vi "Demo - Transient Capture (Multiple Shots)_for_sub_panel.vi"(6 "Soft Trigger":bool=TRUE, 9 "Post-Trigger Samples":i32=100000, 10 "Pre-Trigger Samples":i32, 11 "configuration file path":path) -> ()   [LabVIEW 2017]
doc: "Demonstration of transient capture mode, in a continuos loop"
uses:
  Communications/Communications Library.lvlib
panel:
  in  "stop":bool
  in  "ARM":bool
  out "Waveform Graph":i16[][](graph)
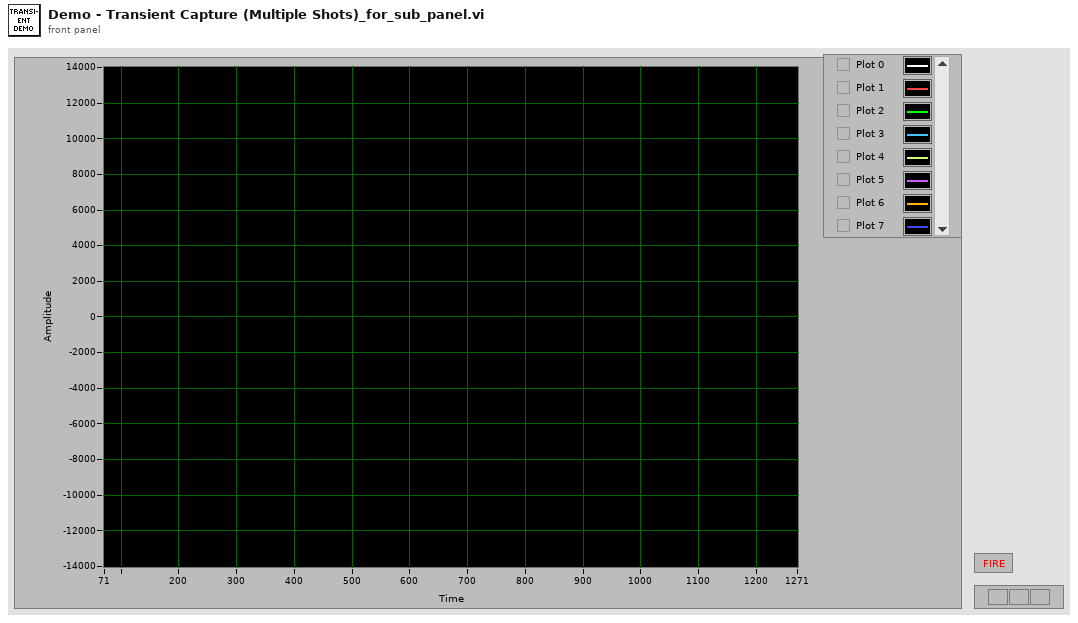
[diagram p1: front panel]
types:
  T1 = typedef "Communications Library.lvlib/DTACQ Module Carrier Configuration--Cluster.ctl" = cluster{"Name":string, "IP":string, "Control Port":i32, "Timeout (ms)":i32, "Continuous Capture Port (Multiplexed)":i32, "Start HIL Shot Port":i32, "AWG Upload Port (Multiplexed)":i32, "Download Captured Data Port (Multiplexed)":i32, "Module Slots":i32, "Module Configurations":T2[]}
  T2 = typedef "Communications Library.lvlib/DTACQ Module Configuration--Cluster.ctl" = cluster{"Name":string, "Position":string, "Module Type":T3, "Control Port":i32, "Timeout (ms)":i32, "Channels":i32}
  T3 = typedef "Communications Library.lvlib/DTACQ Device Type--Enum.ctl" = enum16{"Carrier", "Analog In Module", "Analog Out Module", "Generic Module"}
  T4 = typedef "Communications Library.lvlib/DTACQ Connection Data--Cluster.ctl" = cluster{"Description":string, "Address":string, "Port":u16, "timeout (ms)":i32, "Termination Character":string, "TCP Connection Reference":refnum<k5>, "Open Connection":bool}
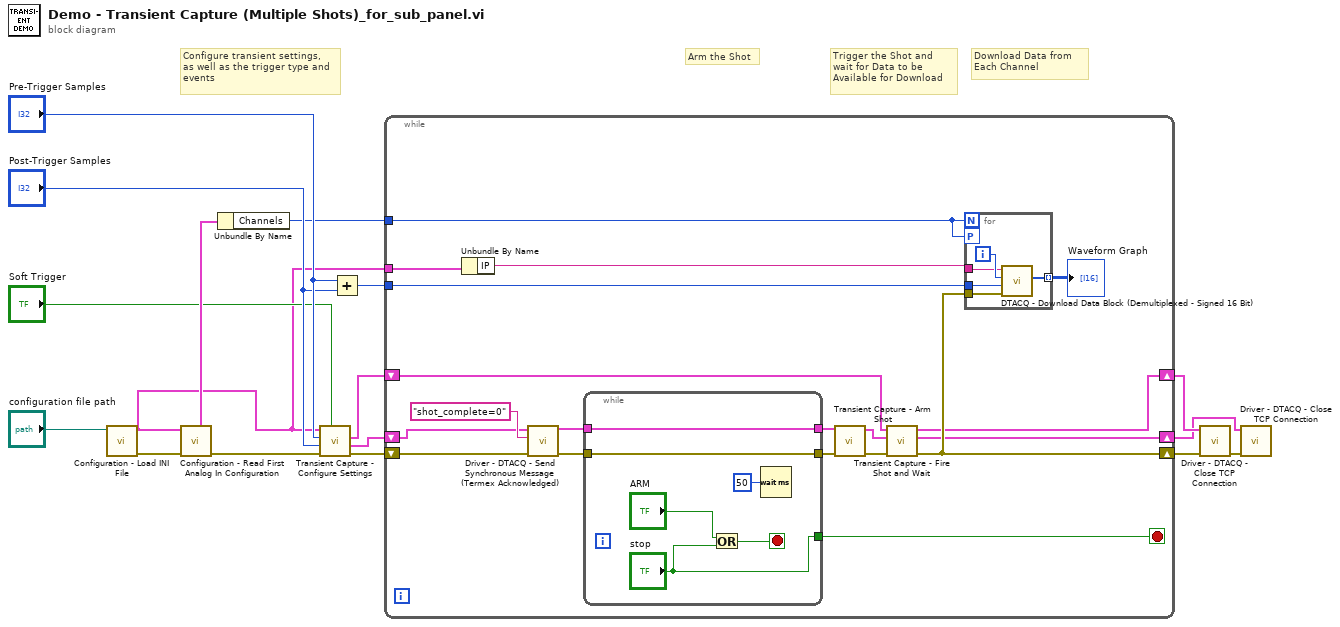
[diagram p0: block diagram]
diagram:
  # "Configure transient settings,\nas well as the trigger type and\nevents"
  # "Trigger the Shot and\nwait for Data to be\nAvailable for Download"
  # "Download Data from \nEach Channel"
  # "Arm the Shot"
  n1 = call "Configuration - Load INI File.vi"("configuration file path"="configuration file path") -> ("error out"=w13:errorcluster, "Carrier Configuration Out"=w1:T1)  [unwired: 9 in]
  n2 = call "Configuration - Read First Analog In Configuration.vi"("error in"=w13, "Carrier Configuration"=w1) -> ("error out"=w12:errorcluster, "AI - Module Configuration"=w14:T2)  [unwired: 5 in, 3 out]
  n3 = Unbundle By Name(w14) -> ("Channels"=w4:i32)
  n4 = call "Transient Capture - Configure Settings.vi"("Soft Trigger"="Soft Trigger", "error in"=w12, "Samples to Read (Post Trigger)"="Post-Trigger Samples", "Samples to Read (Pre Trigger)"="Pre-Trigger Samples", "Carrier Configuration"=w1) -> ("error out"=w10:errorcluster, "Carrier Connection Out"=w3:T4, "AI Connection Out"=w2:T4)  [unwired: 4 in]
  n5 = Add(x="Pre-Trigger Samples", y="Post-Trigger Samples") -> (x+y=w9:i32)
  n6 = while {
    tunnel: w1 -> [w19]
    tunnel: w9 -> [w33]
    tunnel: w4 -> [w25]
    shift-right: [w32] -> w8
    shift-left: w10 -> [w23]
    shift-right: [w31] -> w6
    shift-left: w2 -> [w27]
    shift-right: [w30] -> w5
    shift-left: w3 -> [w22]
    stop <- w26 stop-if-true
    n7 = Unbundle By Name(w19) -> ("IP"=w18:string)
    n8 = call "Driver - DTACQ - Send Synchronous Message (Termex Acknowledged).vi"("error in"=w23, "Message to Send"="shot_complete=0", "DTACQ Connection Data In"=w22) -> ("error out"=w21:errorcluster, "DTACQ Connection Data Out"=w20:T4)  [unwired: 5 in, 2 out]
    n9 = while {
      tunnel: [w38] -> w35
      tunnel: [w37] -> w29
      tunnel: ["stop"] -> w26
      tunnel: w21 -> [w38]
      tunnel: w20 -> [w37]
      stop <- w41 stop-if-true
      n10 = Or(x="ARM", y="stop") -> (x .or. y?=w41:bool)
      n11 = Wait (ms)(milliseconds to wait=u32 50) -> ()  [unwired: 1 out]
    }
    n12 = call "Transient Capture - Arm Shot.vi"("error in"=w35, "Carrier Connection In"=w29) -> ("error out"=w34:errorcluster, "DTACQ Connection Out"=w28:T4)  [unwired: 8 in]
    n13 = call "Transient Capture - Fire Shot and Wait.vi"("error in"=w34, "Carrier Connection In"=w28, "AI Connection In"=w27) -> ("error out"=w32:errorcluster, "Carrier Connection Out"=w30:T4, "AI Connection Out"=w31:T4)  [unwired: 6 in]
    n14 = for {
      N: w25 -> [_]
      tunnel: [w46] -> w36 mode=indexing
      tunnel: w33 -> [w45]
      tunnel: w18 -> [w44]
      tunnel: w32 -> [w43]
      workers-P: w25 -> [_]
      i -> [w47]
      n15 = call "DTACQ - Download Data Block (Demultiplexed - Signed 16 Bit).vi"("error in"=w43, "Maximum Number of Samples"=w45, "Channel Number"=w47, "Address"=w44) -> ("(Signed) 16 Bit Array"=w46:i16[])  [unwired: 5 in, 2 out]
    }
    "Waveform Graph" <- w36
  }
  n16 = call "Driver - DTACQ - Close TCP Connection.vi"("error in"=w8, "DTACQ Connection Data In"=w6) -> ("error out"=w7:errorcluster)  [unwired: 8 in, 1 out]
  n17 = call "Driver - DTACQ - Close TCP Connection.vi"("error in"=w7, "DTACQ Connection Data In"=w5) -> ()  [unwired: 8 in, 2 out]
